vi "Distance from points.vi"(8 "error in (no error)":errorcluster, 10 "Desired Point":cluster{"X":dbl, "Y":dbl}, 11 "Current Point":cluster{"X":dbl, "Y":dbl}) -> (0 "out":errorcluster, 3 "distance":dbl)   [LabVIEW 2017]
panel:
  # "VI Description: Calculates the distance between the current and desired point\nusing distance formula."
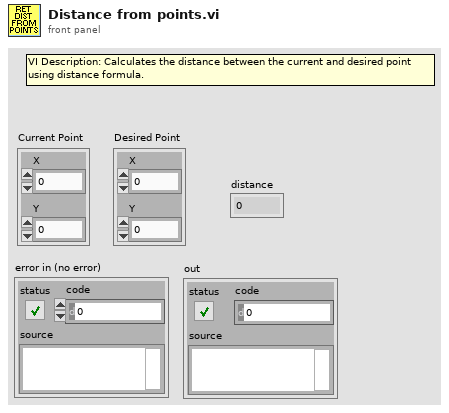
[diagram p1: front panel]
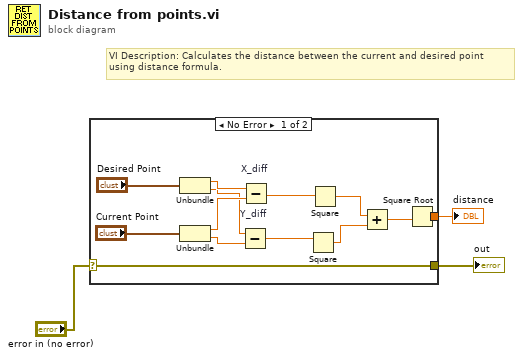
[diagram p0: block diagram]
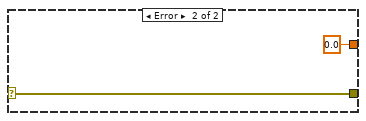
[diagram p2: hidden frame]
diagram:
  # "VI Description: Calculates the distance between the current and desired point\nusing distance formula."
  n1 = case shown="No Error" "error in (no error)" {
    selector: "error in (no error)" -> [w4 w18]
    tunnel: [w5 0.0] -> w3
    tunnel: [w4 w18] -> w1
    frame No Error {
      n2 = Unbundle("Desired Point") -> ("X"=w14:dbl, "Y"=w12:dbl)
      n3 = Unbundle("Current Point") -> ("X"=w13:dbl, "Y"=w11:dbl)
      n4 = Subtract "Y_diff"(x=w12, y=w11) -> (x-y=w9:dbl)
      n5 = Subtract "X_diff"(x=w14, y=w13) -> (x-y=w10:dbl)
      n6 = Square(x=w9) -> (x^2=w7:dbl)
      n7 = Square(x=w10) -> (x^2=w8:dbl)
      n8 = Add(x=w8, y=w7) -> (x+y=w6:dbl)
      n9 = Square Root(x=w6) -> (sqrt(x)=w5:dbl)
    }
    frame Error {
    }
  }
  "distance" <- w3
  "out" <- w1
